vi "Read ConnectionNumber.vi"(8 "error in (no error)":errorcluster, 11 "TCP_Server_Connection_Handler in":refnum<class "TCP_Server_Connection_Handler.lvclass">) -> (0 "error out":errorcluster, 2 "ConnectionNumber":i32, 3 "TCP_Server_Connection_Handler out":refnum<class "TCP_Server_Connection_Handler.lvclass">)   [LabVIEW 2023, in "TCP_Server_Connection_Handler.lvlib" / "TCP_Server_Connection_Handler.lvclass"]
uses:
  TCP_Server_Connection_Handler.lvclass
  TCP_Server_Connection_Handler.lvclass/TCP_Server_Connection_Handler.ctl
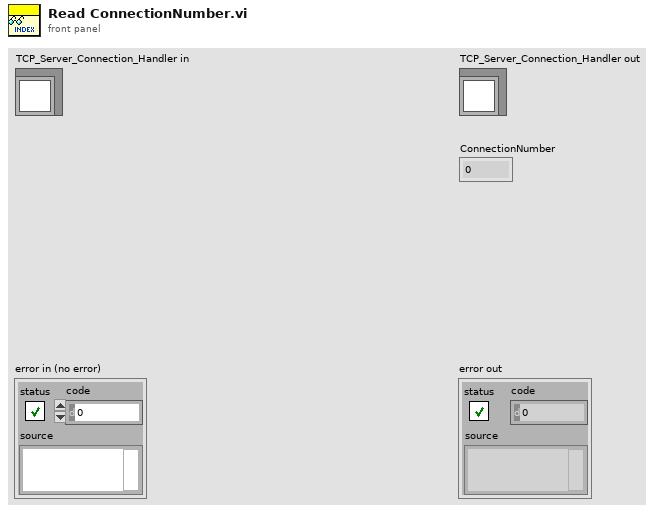
[diagram p1: front panel]
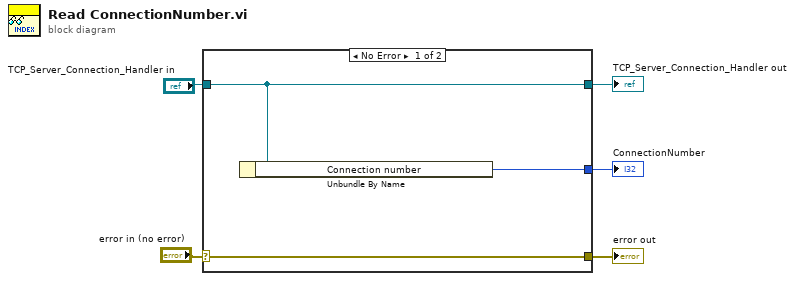
[diagram p0: block diagram]
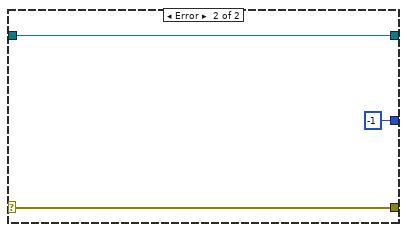
[diagram p2: hidden frame]
diagram:
  n1 = case shown="No Error" "error in (no error)" {
    selector: "error in (no error)" -> [w8 w10]
    tunnel: [w8 w10] -> w4
    tunnel: [w7 w11] -> w2
    tunnel: "TCP_Server_Connection_Handler in" -> [w7 w11]
    tunnel: [w6 -1 ("Connection number")] -> w1
    frame No Error {
      n2 = Unbundle By Name(w7) -> ("Connection number"=w6:i32)
    }
    frame Error {
    }
  }
  "error out" <- w4
  "TCP_Server_Connection_Handler out" <- w2
  "ConnectionNumber" <- w1
